vi "Update Displayed Seconds on Timing.vi"(8 "error in (no error)":errorcluster, 10 "Time(se)":dbl, 11 "Configuration Database in":refnum<class "Configuration Database.lvclass">) -> (0 "error out":errorcluster, 3 "Configuration Database out":refnum<class "Configuration Database.lvclass">)   [LabVIEW 2019, in "Configuration Database Actor.lvlib" / "Configuration Database.lvclass"]
uses:
  Configuration Database.lvclass
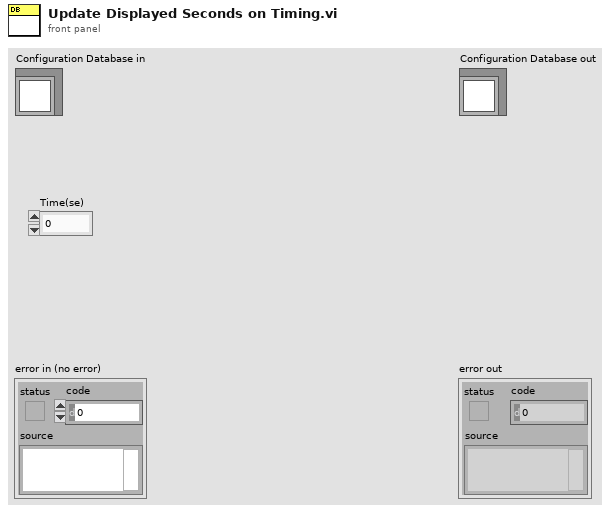
[diagram p1: front panel]
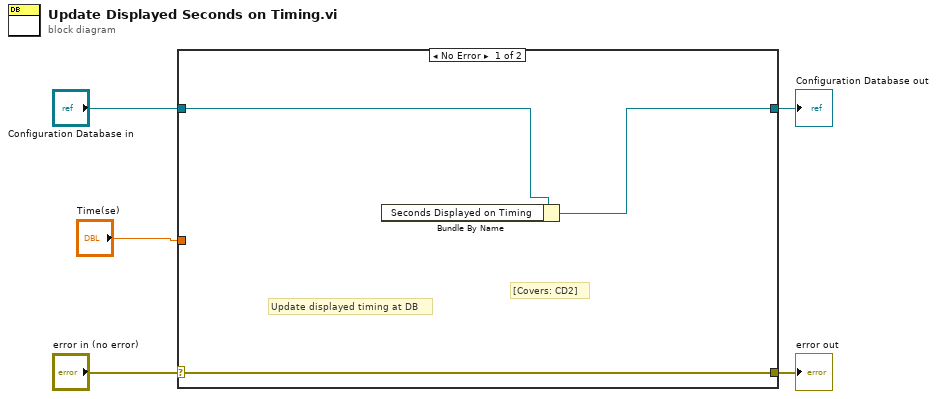
[diagram p0: block diagram]
diagram:
  n1 = case shown="No Error" "error in (no error)" {
    selector: "error in (no error)" -> [w8 w10]
    tunnel: [w8 w10] -> w4
    tunnel: [w6 w9] -> w2
    tunnel: "Configuration Database in" -> [w7 w9]
    tunnel: "Time(se)" -> [_ _]
    frame No Error {
      # "[Covers: CD2]"
      # "Update displayed timing at DB"
      n2 = Bundle By Name(cluster=w7) -> (w6:refnum<class "Configuration Database.lvclass">)  [unwired: 1 in]
    }
    frame Error {
    }
  }
  "error out" <- w4
  "Configuration Database out" <- w2
